vi "Create Single Serial Channel Resources.vi"() -> (4 "single serial channel resources":T1)   [LabVIEW 2021, in "GettingStarted_Common_148X_FPGA.lvlib"]
uses:
  GettingStarted_Common_148X_FPGA.lvlib
  Types/Single Serial Channel Resources.ctl
  <vilib>/rvi/DataTransferAndStorage/Container/Common/niFpgaContainerGetUniqueNameForEmu.vi
  <vilib>/rvi/DataTransferAndStorage/Container/Common/niFpgaContainerSetEmuInfo.vi
  <vilib>/rvi/eio/common/nirviEmuReportErrorAndStop.vi
  <vilib>/rvi/LocalResourceManager/LocalResourceManager.xnode
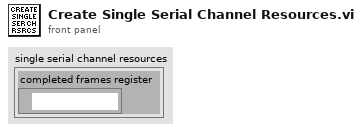
[diagram p1: front panel]
types:
  T1 = typedef "GettingStarted_Common_148X_FPGA.lvlib/Single Serial Channel Resources.ctl" = cluster{"completed frames register":refnum<k21>}
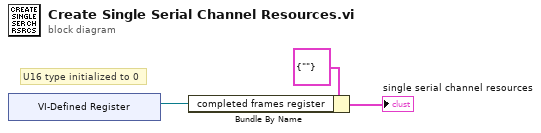
[diagram p0: block diagram]
diagram:
  # "U16 type initialized to 0"
  n1 = xnode "VI-Defined Register"() -> ("Register Out"=w2:refnum<k21>)
  n2 = Bundle By Name(cluster=T1 {"completed frames register"=""} ("serial channel data resources"), "completed frames register"=w2) -> (→"single serial channel resources":T1)
